vi "winForms initSyntaxColoring.vi"(5 "editorType":T1, 6 "error in (no error)":errorcluster, 9 "scintillaRefNum in":refnum<k24>) -> (0 "error out":errorcluster, 3 "scintillaRefNum out":refnum<k24>)   [LabVIEW 2018]
uses:
  C:/ATI_MS_InstrumentControl/dll/ScintillaNET.dll
  dll/ScintillaNET.dll
  winForms editorType.ctl
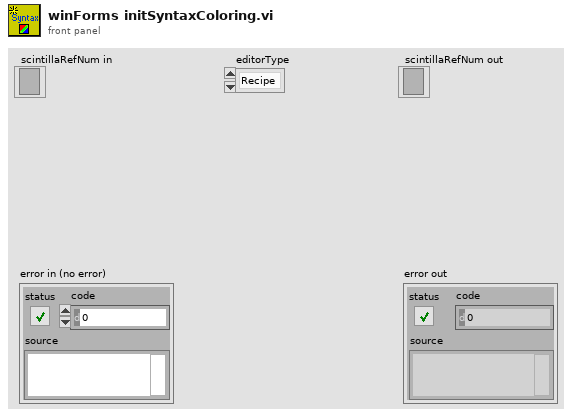
[diagram p1: front panel]
types:
  T1 = typedef "winForms editorType.ctl" = enum16{"Recipe", "SigProc", "Editor"}
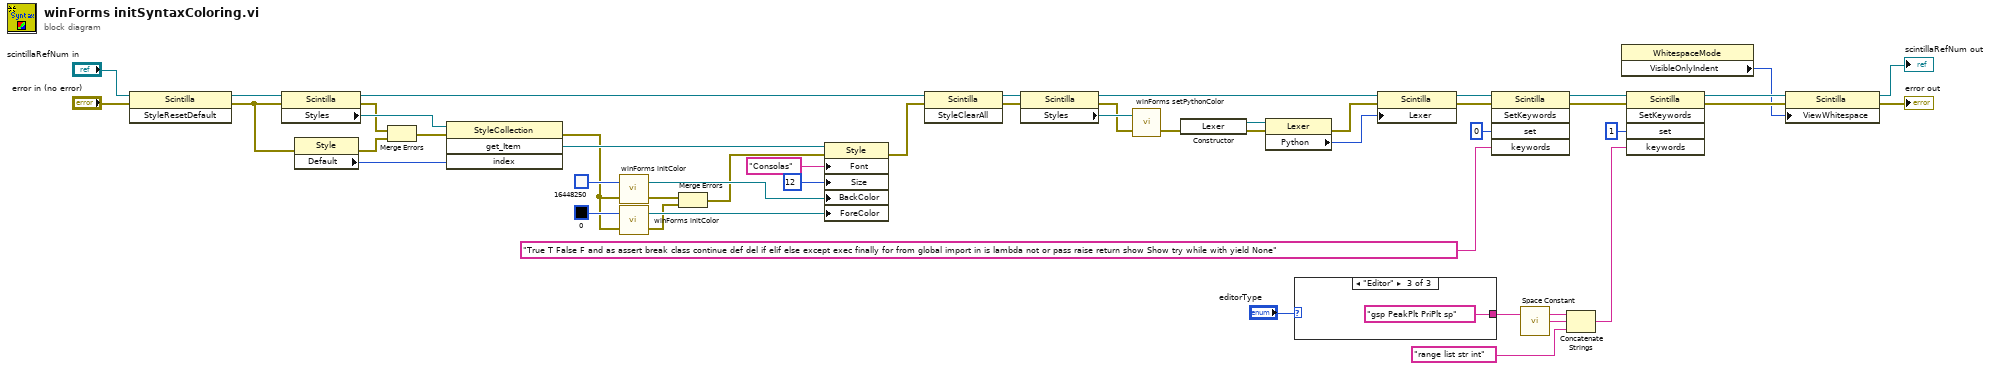
[diagram p0: block diagram]
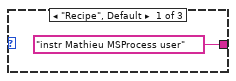
[diagram p2: hidden frame]
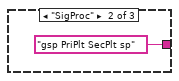
[diagram p3: hidden frame]
diagram:
  n1 = invoke class="Scintilla" method="StyleResetDefault"(reference="scintillaRefNum in", error in="error in (no error)") -> (reference out=w46:refnum<k24>, error out=w27:errorcluster)  [unwired: 1 in, 1 out]
  n2 = property class="Scintilla"(reference=w46, error in=w27) -> (reference out=w36:refnum<k24>, error out=w25:errorcluster, "Styles"=w45:refnum<k24>)
  n3 = property class="Style"(error in=w27) -> (error out=w26:errorcluster, "Default"=w44:i32)  [unwired: 1 in, 1 out]
  n4 = Merge Errors(w25, w26) -> (w24:errorcluster)
  n5 = invoke class="StyleCollection" method="get_Item"(reference=w45, error in=w24, "index"=w44) -> (error out=w21:errorcluster, "get_Item"=w43:refnum<k24>)  [unwired: 1 in, 2 out]
  n6 = call "winForms initColor.vi"("error in (no error)"=w21, "Color Box"=u32 16448250) -> ("error out"=w20:errorcluster, "reference out"=w37:refnum<k24>)
  n7 = call "winForms initColor.vi"("error in (no error)"=w21, "Color Box"=u32 0) -> ("error out"=w19:errorcluster, "reference out"=w38:refnum<k24>)
  n8 = Merge Errors(w20, w19) -> (w18:errorcluster)
  n9 = property class="Style"(reference=w43, error in=w18, "Font"="Consolas", "Size"=12, "BackColor"=w37, "ForeColor"=w38) -> (error out=w35:errorcluster)  [unwired: 1 out]
  n10 = invoke class="Scintilla" method="StyleClearAll"(reference=w36, error in=w35) -> (reference out=w34:refnum<k24>, error out=w33:errorcluster)  [unwired: 1 in, 1 out]
  n11 = property class="Scintilla"(reference=w34, error in=w33) -> (reference out=w32:refnum<k24>, error out=w23:errorcluster, "Styles"=w30:refnum<k24>)
  n12 = call "winForms setPythonColor.vi"("error in (no error)"=w23, "stylesRefNum"=w30) -> ("error out"=w29:errorcluster)  [unwired: 1 in]
  n13 = constructor class="Lexer"(error in=w29) -> (reference out=w48:refnum<k24>, error out=w47:errorcluster)  [unwired: 2 in, 1 out]
  n14 = property class="Lexer"(reference=w48, error in=w47) -> (error out=w22:errorcluster, "Python"=w31:i32)  [unwired: 1 out]
  n15 = case shown="\"Editor\"" "editorType" {
    tunnel: ["instr Mathieu MSProcess user" ("keywords") "gsp PriPlt SecPlt sp" ("keywords") "gsp PeakPlt PriPlt sp" ("keywords")] -> w3
    frame "Recipe", Default {
    }
    frame "SigProc" {
    }
    frame "Editor" {
    }
  }
  n16 = property class="Scintilla"(reference=w32, error in=w22, "Lexer"=w31) -> (reference out=w17:refnum<k24>, error out=w14:errorcluster)
  n17 = invoke class="Scintilla" method="SetKeywords"(reference=w17, error in=w14, "set"=0, "keywords"="True T False F and as assert break class continue def del if elif else except exec finally for from global import in is lambda not or pass raise return show Show try while with yield None") -> (reference out=w13:refnum<k24>, error out=w12:errorcluster)  [unwired: 1 in, 3 out]
  n18 = call <vilib>:"Space Constant.vi"() -> ("String"=w4:string)
  n19 = Concatenate Strings(w3, w4, "range list str int") -> (w1:string)
  n20 = property class="WhitespaceMode"() -> ("VisibleOnlyIndent"=w8:i32)  [unwired: 2 in, 2 out]
  n21 = invoke class="Scintilla" method="SetKeywords"(reference=w13, error in=w12, "set"=1, "keywords"=w1) -> (reference out=w10:refnum<k24>, error out=w9:errorcluster)  [unwired: 1 in, 3 out]
  n22 = property class="Scintilla"(reference=w10, error in=w9, "ViewWhitespace"=w8) -> (reference out=→"scintillaRefNum out":refnum<k24>, error out=→"error out":errorcluster)
